vi "Parse Formula Node.vi"(2 "error in (no error)":errorcluster, 3 "formula":string, 4 "Variables Output":string[](array[string]), 5 "Variables Input":string[](array[string])) -> (0 "error out":errorcluster, 1 "Parsed Formula Node":T1 {"Y Values" format="%.2f"})   [LabVIEW 2010, in "NI_Gmath.lvlib"]
doc: "Analyzes Eval Formula Node VI inputs and yields an intermediate state as an input for the Eval Parsed Formula Node VI."
uses:
  NI_Gmath.lvlib
panel:
  # "Example:\n\n Variables Input: a and b\n Variables Output: x and y \n formula: x=a+b;y=a*b;"
  # "operator"
  # "register1"
  # "register2"
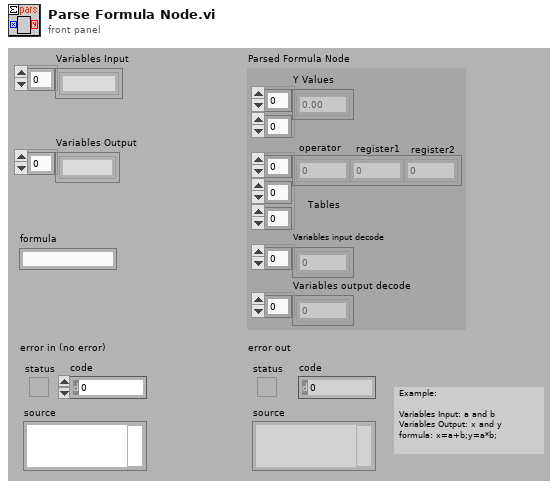
[diagram p1: front panel]
types:
  T1 = cluster{"Y Values":dbl[][], "Tables":i32[][][], "Variables input decode":i32[], "Variables output decode":i32[]}
  T2 = cluster{"Y Values":dbl[][], "Table":i32[][][], i32[], i32[]}
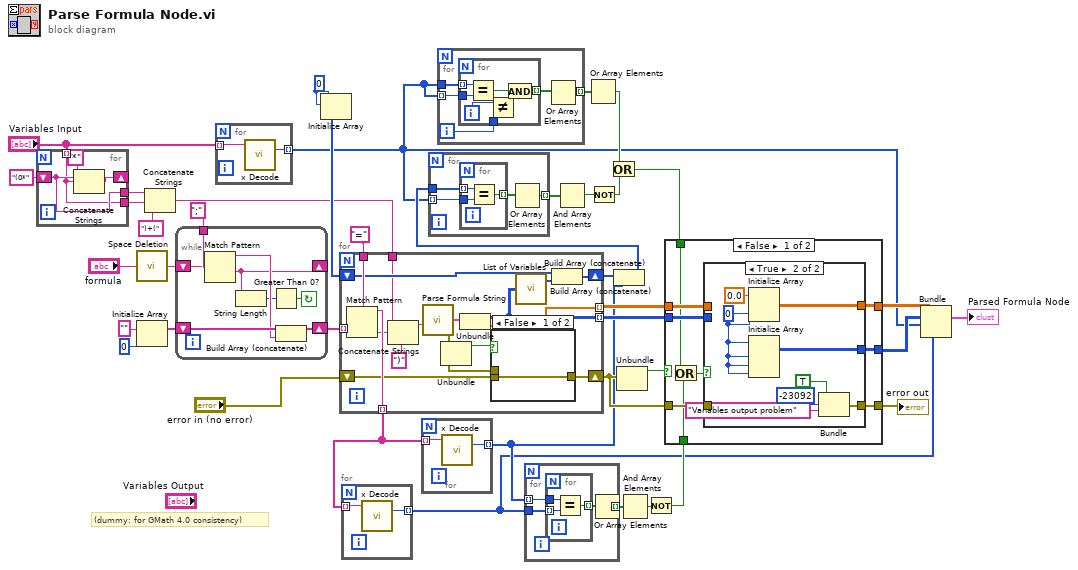
[diagram p0: block diagram]
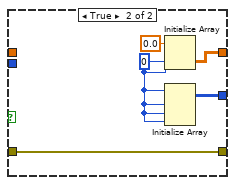
[diagram p3: hidden frame]
diagram:
  w26 = 0
  # "(dummy: for GMath 4.0 consistency)"
  n1 = for {
    shift-right: [w43] -> _
    shift-left: "(0*" -> [w42]
    tunnel: "Variables Input" -> [w41] mode=indexing
    tunnel: [w42] -> w10
    tunnel: [w41] -> w9
    n2 = Concatenate Strings(w42, w41, "*") -> (w43:string)
  }
  n3 = call "Space Deletion.vi"("string with spaces"="formula") -> ("string without spaces"=w36:string)
  n4 = Initialize Array("", 0) -> (w37:string[])
  n5 = Concatenate Strings(w10, w9, ")+(") -> (w6:string)
  n6 = while {
    shift-left: w36 -> [w48]
    shift-right: [w45] -> _
    shift-left: w37 -> [w52]
    shift-right: [w51] -> w34
    tunnel: ";" -> [w50]
    stop <- w46 continue-if-true
    n7 = Match Pattern(string=w48, regular expression=w50) -> (before substring=w49:string, after substring=w45:string)  [unwired: 1 in, 2 out]
    n8 = String Length(string=w45) -> (length=w47:i32)
    n9 = Greater Than 0?(x=w47) -> (x > 0?=w46:bool)
    n10 = Build Array (concatenate)(w52, w49) -> (w51:string[])
  }
  n11 = for {
    tunnel: "Variables Input" -> [w54] mode=indexing
    tunnel: [w53] -> w14 mode=indexing
    n12 = call "x Decode.vi"("x string"=w54) -> ("number"=w53:i32)  [unwired: 1 in, 1 out]
  }
  n13 = Initialize Array(w26, w26) -> (w25:i32[])
  n14 = for {
    tunnel: "=" -> [w71]
    tunnel: w34 -> [w70] mode=indexing
    tunnel: [w60] -> w31 mode=indexing
    tunnel: [w59] -> w32 mode=indexing
    tunnel: [w69] -> w5 mode=indexing
    shift-right: [w65] -> w30
    shift-left: "error in (no error)" -> [w66]
    shift-right: [w62] -> w23
    shift-left: w25 -> [w64]
    tunnel: w6 -> [w57]
    n15 = Match Pattern(string=w70, regular expression=w71) -> (before substring=w69:string, after substring=w56:string)  [unwired: 1 in, 2 out]
    n16 = Concatenate Strings(w57, w56, ")") -> (w55:string)
    n17 = call "Parse Formula String.vi"("formula"=w55) -> ("error out"=w68:errorcluster, "Parsed Formula"=w61:cluster{"Table":i32[][], "Y Values":dbl[]})  [unwired: 1 in]
    n18 = Unbundle(w68) -> ("status"=w67:bool)  [unwired: 2 out]
    n19 = Unbundle(w61) -> ("Table"=w60:i32[][], "Y Values"=w59:dbl[])
    n20 = case shown="False" w67 {
      tunnel: w66 -> [w72 _]
      tunnel: [w72 w73] -> w65
      tunnel: w68 -> [_ w73]
      frame False {
      }
      frame True {
      }
    }
    n21 = call "List of Variables.vi"("Table"=w60) -> ("List of variables"=w63:i32[])
    n22 = Build Array (concatenate)(w64, w63) -> (w62:i32[])
  }
  n23 = for {
    tunnel: w5 -> [w75] mode=indexing
    tunnel: [w74] -> w4 mode=indexing
    n24 = call "x Decode.vi"("x string"=w75) -> ("number"=w74:i32)  [unwired: 1 in, 1 out]
  }
  n25 = for {
    tunnel: w5 -> [w77] mode=indexing
    tunnel: [w76] -> w17 mode=indexing
    n26 = call "x Decode.vi"("x string"=w77) -> ("number"=w76:i32)  [unwired: 1 in, 1 out]
  }
  n27 = for {
    tunnel: w14 -> [w82] mode=indexing
    tunnel: w14 -> [w81]
    tunnel: [w79] -> w21 mode=indexing
    i -> [w78]
    n28 = for {
      tunnel: w82 -> [w89]
      tunnel: w81 -> [w88] mode=indexing
      tunnel: [w83] -> w80 mode=indexing
      tunnel: w78 -> [w86]
      i -> [w87]
      n29 = Equal?(x=w88, y=w89) -> (x = y?=w84:bool)
      n30 = Not Equal?(x=w87, y=w86) -> (x != y?=w85:bool)
      n31 = And(x=w84, y=w85) -> (x .and. y?=w83:bool)
    }
    n32 = Or Array Elements(Boolean array=w80) -> (logical OR=w79:bool)
  }
  n33 = for {
    tunnel: w4 -> [w93]
    tunnel: w17 -> [w92] mode=indexing
    tunnel: [w90] -> w29 mode=indexing
    n34 = for {
      tunnel: w93 -> [w96] mode=indexing
      tunnel: w92 -> [w95]
      tunnel: [w94] -> w91 mode=indexing
      n35 = Equal?(x=w95, y=w96) -> (x = y?=w94:bool)
    }
    n36 = Or Array Elements(Boolean array=w91) -> (logical OR=w90:bool)
  }
  n37 = Or Array Elements(Boolean array=w21) -> (logical OR=w19:bool)
  n38 = Build Array (concatenate)(w23, w17) -> (w22:i32[])
  n39 = for {
    tunnel: w14 -> [w100] mode=indexing
    tunnel: w22 -> [w99]
    tunnel: [w97] -> w24 mode=indexing
    n40 = for {
      tunnel: w100 -> [w103]
      tunnel: w99 -> [w102] mode=indexing
      tunnel: [w101] -> w98 mode=indexing
      n41 = Equal?(x=w102, y=w103) -> (x = y?=w101:bool)
    }
    n42 = Or Array Elements(Boolean array=w98) -> (logical OR=w97:bool)
  }
  n43 = And Array Elements(Boolean array=w24) -> (logical AND=w27:bool)
  n44 = Not(x=w27) -> (.not. x?=w13:bool)
  n45 = Or(x=w19, y=w13) -> (x .or. y?=w20:bool)
  n46 = Unbundle(w30) -> ("status"=w33:bool)  [unwired: 2 out]
  n47 = And Array Elements(Boolean array=w29) -> (logical AND=w28:bool)
  n48 = Not(x=w28) -> (.not. x?=w18:bool)
  n49 = case shown="False" w33 {
    tunnel: [w112 w126] -> w16
    tunnel: [w111 w125] -> w15
    tunnel: w18 -> [w104 _]
    tunnel: w32 -> [w110 _]
    tunnel: w31 -> [w109 _]
    tunnel: w30 -> [w108 w124]
    tunnel: [w107 w124] -> w2
    tunnel: w20 -> [w105 _]
    frame False {
      n50 = Or(x=w105, y=w104) -> (x .or. y?=w106:bool)
      n51 = case shown="True" w106 {
        tunnel: [w115 w121] -> w112
        tunnel: [w114 w120] -> w111
        tunnel: w110 -> [w115 _]
        tunnel: w109 -> [w114 _]
        tunnel: w108 -> [w113 _]
        tunnel: [w113 w119] -> w107
        frame False {
        }
        frame True {
          w123 = 0
          n52 = Initialize Array(0.0, w123, w123) -> (w121:dbl[][])
          n53 = Initialize Array(w123, w123, w123, w123) -> (w120:i32[][][])
          n54 = Bundle(TRUE, -23092, "Variables output problem") -> (w119:errorcluster)  [unwired: 1 in]
        }
      }
    }
    frame True {
      w128 = 0
      n55 = Initialize Array(0.0, w128, w128) -> (w126:dbl[][])
      n56 = Initialize Array(w128, w128, w128, w128) -> (w125:i32[][][])
    }
  }
  "error out" <- w2
  n57 = Bundle("Y Values"=w16, "Table"=w15, w14, w4) -> (→"Parsed Formula Node":T2)  [unwired: 1 in]
